vi "LPS22HH Temp. Calc..vi"(10 "TEMP_OUT_L":u32[](array[numeric]), 11 "TEMP_OUT_H":u32[](array[numeric])) -> (3 "Thermometer":dbl(slide) scale=0.0..40.0)   [LabVIEW 2020, in "LPS22Demo.lvlib"]
uses:
  LPS22Demo.lvlib
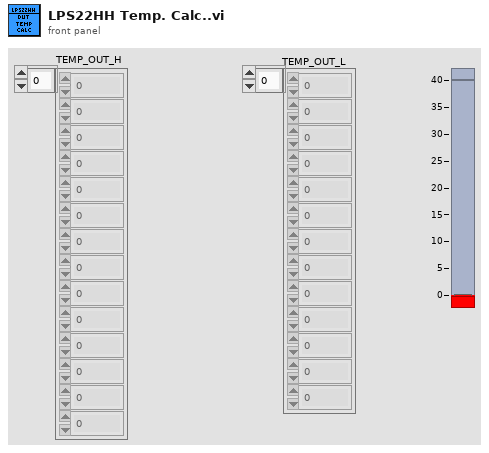
[diagram p1: front panel]
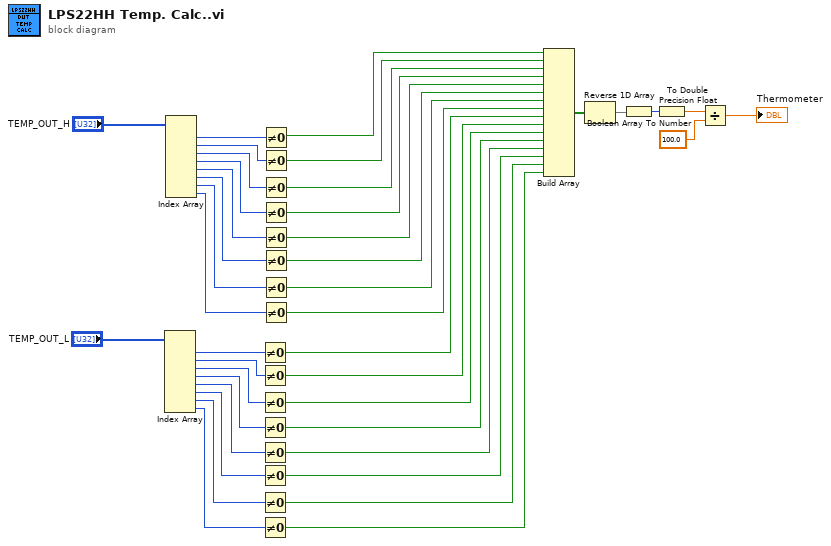
[diagram p0: block diagram]
diagram:
  n1 = Index Array(array="TEMP_OUT_L") -> (element #1=w15:u32, element #2=w23:u32, element #3=w22:u32, element #4=w21:u32, element #5=w20:u32, element #6=w19:u32, element #7=w18:u32, element #8=w17:u32)  [unwired: 8 in]
  n2 = Index Array(array="TEMP_OUT_H") -> (element #1=w32:u32, element #2=w40:u32, element #3=w39:u32, element #4=w38:u32, element #5=w37:u32, element #6=w36:u32, element #7=w35:u32, element #8=w34:u32)  [unwired: 8 in]
  n3 = Not Equal To 0?(x=w15) -> (x != 0?=w14:bool)
  n4 = Not Equal To 0?(x=w23) -> (x != 0?=w13:bool)
  n5 = Not Equal To 0?(x=w22) -> (x != 0?=w12:bool)
  n6 = Not Equal To 0?(x=w21) -> (x != 0?=w11:bool)
  n7 = Not Equal To 0?(x=w20) -> (x != 0?=w10:bool)
  n8 = Not Equal To 0?(x=w19) -> (x != 0?=w9:bool)
  n9 = Not Equal To 0?(x=w18) -> (x != 0?=w8:bool)
  n10 = Not Equal To 0?(x=w17) -> (x != 0?=w7:bool)
  n11 = Not Equal To 0?(x=w32) -> (x != 0?=w31:bool)
  n12 = Not Equal To 0?(x=w40) -> (x != 0?=w30:bool)
  n13 = Not Equal To 0?(x=w39) -> (x != 0?=w29:bool)
  n14 = Not Equal To 0?(x=w38) -> (x != 0?=w28:bool)
  n15 = Not Equal To 0?(x=w37) -> (x != 0?=w27:bool)
  n16 = Not Equal To 0?(x=w36) -> (x != 0?=w26:bool)
  n17 = Not Equal To 0?(x=w35) -> (x != 0?=w25:bool)
  n18 = Not Equal To 0?(x=w34) -> (x != 0?=w24:bool)
  n19 = Build Array(w31, w30, w29, w28, w27, w26, w25, w24, w14, w13, w12, w11, w10, w9, w8, w7) -> (w6:bool[])
  n20 = Reverse 1D Array(array=w6) -> (reversed array=w5:bool[])
  n21 = Boolean Array To Number(Boolean array=w5) -> (number=w2:u32)
  n22 = To Double Precision Float(number=w2) -> (double precision float=w1:dbl)
  n23 = Divide(x=w1, y=100.0) -> (x/y=→"Thermometer":dbl)
